vi "tlc_Cue Module.vi"(5 "Number of Channels":cluster{"Rows":i32, "Columns":i32}, 6 "Command":T3, 7 "error in (no error)":errorcluster, 8 "Cue Input":T1={"Cue Name"="", "Wait Time (s)"=0, "Fade Time (s)"=1, "Follow Time (s)"=0, "Channels"=[]} {"Channels"."Intensity" min=0.0 max=100.0 step=1.0 format="%#.0f"}, 10 "Cue Index":i32 min=0) -> (0 "error out":errorcluster, 1 "Cue Output":T1 {"Channels"."Intensity" min=0.0 max=100.0 step=1.0 format="%#.0f"}, 2 "Number of Cues":i32)   [LabVIEW 2009]
doc: "[Covers: REQ_MinimumChannels]\nControls access to the Cue data."
uses:
  tlc_Cue_Information Command.ctl
  Controls/tlc_Cue_Information.ctl
  Controls/channel.ctl
panel:
  # "Output"
  # "Input"
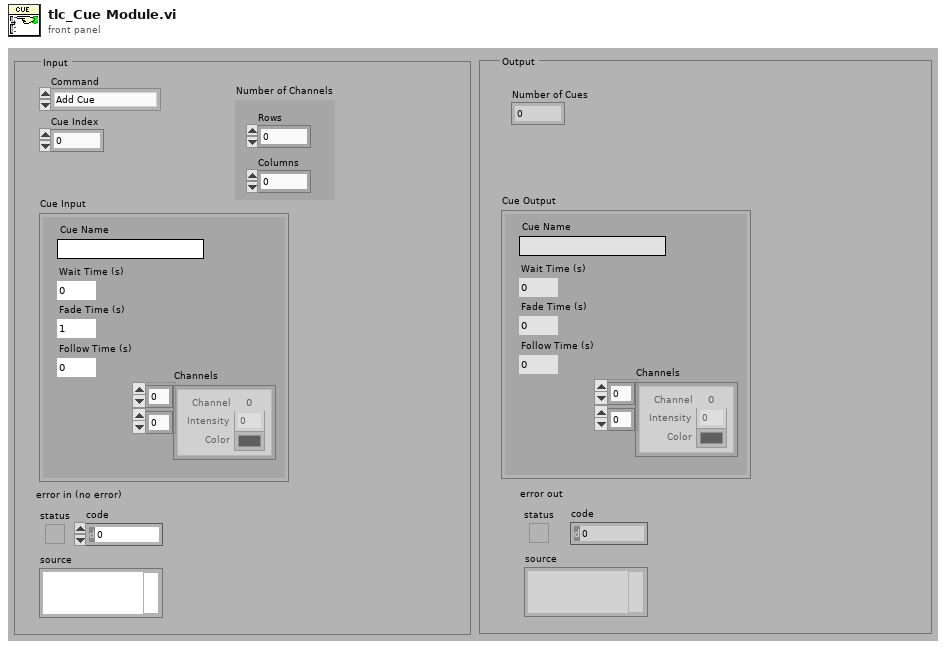
[diagram p1: front panel]
types:
  T1 = typedef "tlc_Cue_Information.ctl" = cluster{"Cue Name":string, "Wait Time (s)":u32, "Fade Time (s)":u32, "Follow Time (s)":u32, "Channels":T2[][]}
  T2 = typedef "channel.ctl" = cluster{"Intensity":dbl, " Color":u32, "Channel":i32}
  T3 = typedef "tlc_Cue_Information Command.ctl" = enum16{"Add Cue", "Get Cue Values", "Set Cue Values", "Get Number of Cues", "Initialize", "Get Empty Cue"}
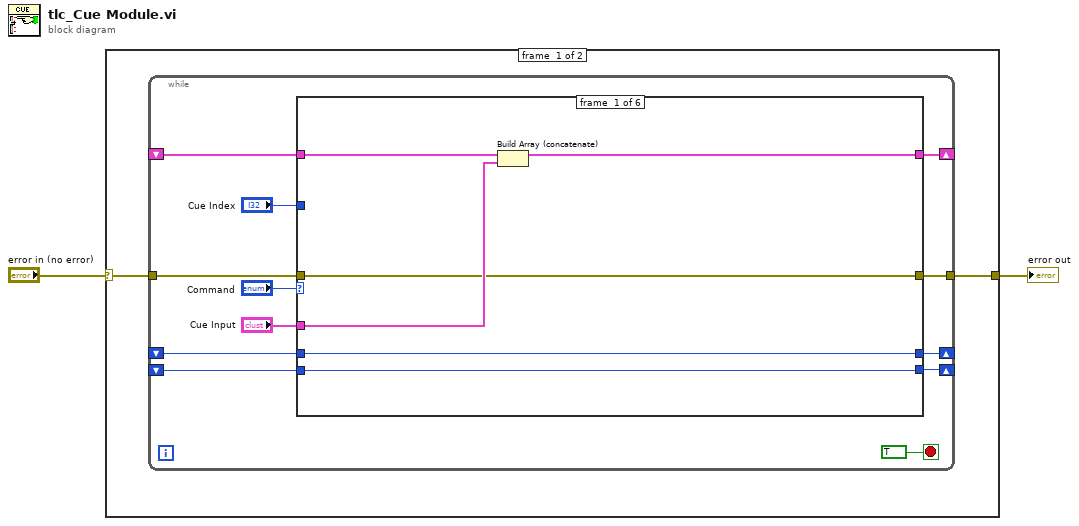
[diagram p0: block diagram]
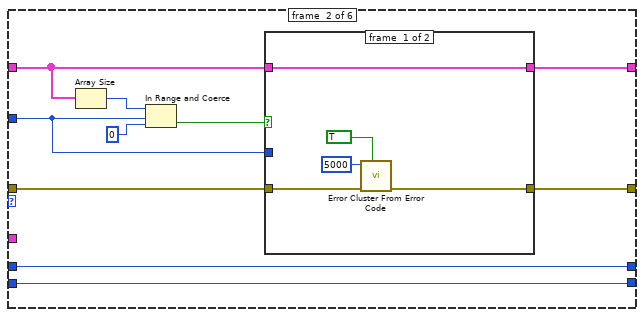
[diagram p2: hidden frame]
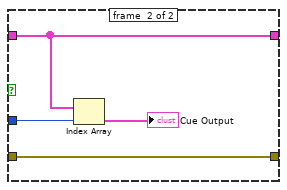
[diagram p3: hidden frame]
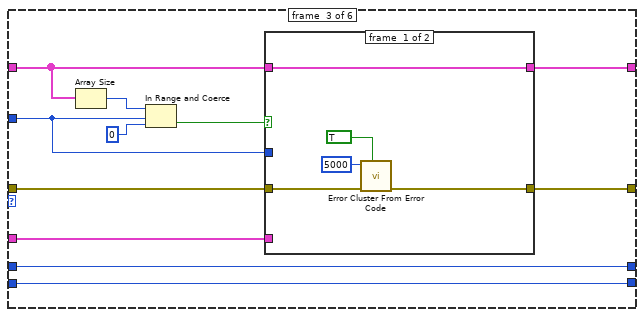
[diagram p4: hidden frame]
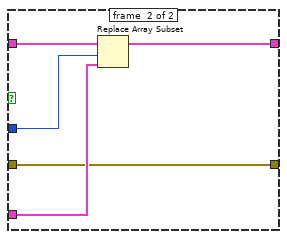
[diagram p5: hidden frame]
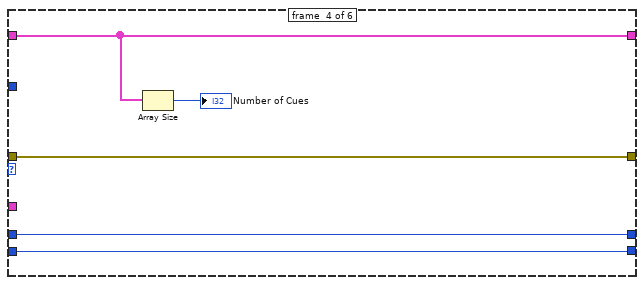
[diagram p6: hidden frame]
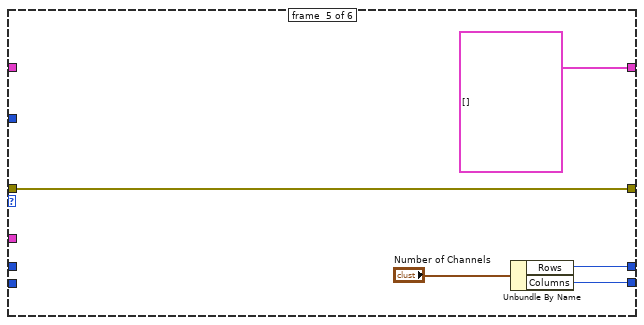
[diagram p7: hidden frame]
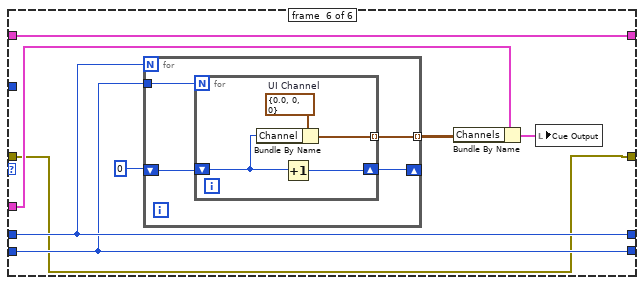
[diagram p8: hidden frame]
diagram:
  n1 = case shown="No Error" "error in (no error)" {
    selector: "error in (no error)" -> [w4 w89]
    tunnel: [w3 w89] -> w1
    frame #0 {
      n2 = while {
        shift-right: [w13] -> _
        shift-left: _ -> [w12]
        shift-right: [w10] -> _
        shift-left: _ -> [w8]
        shift-right: [w9] -> _
        shift-left: _ -> [w7]
        tunnel: w4 -> [w6]
        tunnel: [w5] -> w3
        stop <- TRUE stop-if-true
        n3 = case shown="\"Get Cue Values\"" "Command" {
          tunnel: "Cue Input" -> [w22 _ w51 _ _ w74]
          tunnel: [w21 w27 w52 w67 T1[] [] w77] -> w13
          tunnel: w12 -> [w20 w30 w47 w67 _ w77]
          tunnel: "Cue Index" -> [_ w24 w43 _ _ _]
          tunnel: [w19 w32 w50 w65 w70 w80] -> w10
          tunnel: [w18 w31 w49 w64 w69 w79] -> w9
          tunnel: w8 -> [w19 w32 w50 w65 _ w80]
          tunnel: w7 -> [w18 w31 w49 w64 _ w79]
          tunnel: [w17 w25 w46 w63 w68 w73] -> w5
          tunnel: w6 -> [w17 w26 w45 w63 w68 w73]
          frame #0 {
            n4 = Build Array (concatenate) "Build Array"(w20, w22) -> (w21:T1[])
          }
          frame #1 {
            n5 = Array Size(array=w30) -> (size(s)=w23:i32)
            n6 = In Range and Coerce(upper limit=w23, x=w24, lower limit=0) -> (In Range?=w28:bool)  [unwired: 1 out]
            n7 = case shown="False" w28 {
              tunnel: w30 -> [w37 w40]
              tunnel: [w37 w40] -> w27
              tunnel: w26 -> [w36 w39]
              tunnel: [w35 w39] -> w25
              tunnel: w24 -> [_ w38]
              frame #0 {
                n8 = call <vilib>:"Error Cluster From Error Code.vi"("show call chain? (False)"=TRUE, "error in (no error)"=w36, "error code (0)"=5000) -> ("error out"=w35:errorcluster)  [unwired: 6 in]
              }
              frame #1 {
                n9 = Index Array "Index Array"(array=w40, index=w38) -> (element=→"Cue Output":T1)
              }
            }
          }
          frame #2 {
            n10 = Array Size(array=w47) -> (size(s)=w42:i32)
            n11 = In Range and Coerce(upper limit=w42, x=w43, lower limit=0) -> (In Range?=w44:bool)  [unwired: 1 out]
            n12 = case shown="False" w44 {
              tunnel: [w53 w62] -> w52
              tunnel: w51 -> [_ w61]
              tunnel: w47 -> [w53 w60]
              tunnel: [w54 w59] -> w46
              tunnel: w45 -> [w55 w59]
              tunnel: w43 -> [_ w58]
              frame #0 {
                n13 = call <vilib>:"Error Cluster From Error Code.vi"("show call chain? (False)"=TRUE, "error in (no error)"=w55, "error code (0)"=5000) -> ("error out"=w54:errorcluster)  [unwired: 6 in]
              }
              frame #1 {
                n14 = Replace Array Subset "Replace Array Subset"(array=w60, new element=w61, index=w58) -> (w62:T1[])
              }
            }
          }
          frame #3 {
            n15 = Array Size(array=w67) -> (size(s)=→"Number of Cues":i32)
          }
          frame #4 {
            n16 = Unbundle By Name("Number of Channels") -> ("Rows"=w70:i32, "Columns"=w69:i32)
          }
          frame #5 {
            n17 = for {
              N: w80 -> [_]
              tunnel: w79 -> [w84]
              shift-right: [w81] -> _
              shift-left: 0 -> [w83]
              tunnel: [w82] -> w76 mode=indexing
              n18 = for {
                N: w84 -> [_]
                shift-right: [w87] -> w81
                shift-left: w83 -> [w86]
                tunnel: [w85] -> w82 mode=indexing
                w88 = T2 {"Intensity"=0.0, " Color"=0, "Channel"=0}  # UI Channel
                n19 = Bundle By Name "Bundle By Name"(cluster=w88, "Channel"=w86) -> (w85:T2)
                n20 = Increment(x=w86) -> (x+1=w87:i32)
              }
            }
            n21 = Bundle By Name "Bundle By Name"(cluster=w74, "Channels"=w76) -> (w75:T1)
            n22 = local write "Cue Output"(w75) -> ()
          }
        }
      }
    }
    frame #1 {
    }
  }
  "error out" <- w1
